vi "create backup files.vi"(8 "error in (no error)":errorcluster caption="错误输入（无错误）", 10 "execute file name":string, 11 "路径":path) -> (0 "error out":errorcluster caption="错误输出")   [LabVIEW 2016, in "数据传输系统-04.lvlib" / "update.lvlib"]
uses:
  update.lvlib
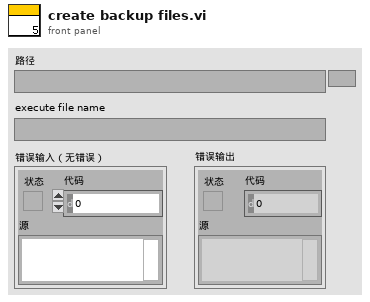
[diagram p1: front panel]
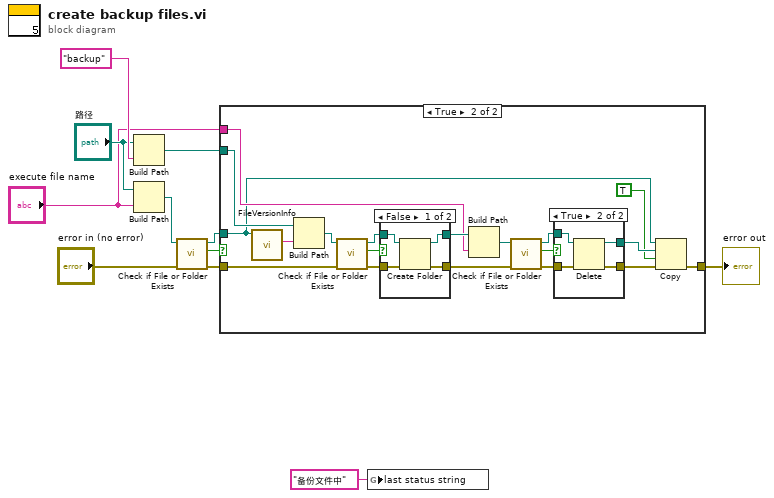
[diagram p0: block diagram]
diagram:
  n1 = Build Path(base path="路径", name or relative path="backup" ("名称或相对路径")) -> (appended path=w10:path)
  n2 = Build Path(base path="路径", name or relative path="execute file name") -> (appended path=w6:path)
  n3 = call <vilib>:"Check if File or Folder Exists.vi"("error in (no error)"="error in (no error)", "path"=w6) -> ("error out"=w3:errorcluster, "file or folder exists?"=w5:bool, "dup path"=w2:path)  [unwired: 7 in]
  n4 = case shown="True" w5 {
    tunnel: w3 -> [w12 w22]
    tunnel: w10 -> [_ w21]
    tunnel: "execute file name" -> [_ w18]
    tunnel: [w12 w14] -> w7
    tunnel: w2 -> [_ w13]
    frame False {
    }
    frame True {
      n5 = call <vilib>:"FileVersionInfo.vi"("Application Path in"=w13) -> ("File Version Info"=w20:string)  [unwired: 7 in, 3 out]
      n6 = Build Path(base path=w21, name or relative path=w20) -> (appended path=w19:path)
      n7 = call <vilib>:"Check if File or Folder Exists.vi"("error in (no error)"=w22, "path"=w19) -> ("error out"=w24:errorcluster, "file or folder exists?"=w31:bool, "dup path"=w30:path)  [unwired: 7 in]
      n8 = case shown="False" w31 {
        tunnel: w30 -> [w41 w43]
        tunnel: [w40 w43] -> w29
        tunnel: w24 -> [w39 w42]
        tunnel: [w38 w42] -> w23
        frame False {
          n9 = Create Folder(path (use dialog)=w41, error in=w39) -> (created path=w40:path, error out=w38:errorcluster)  [unwired: 1 in, 1 out]
        }
        frame True {
        }
      }
      n10 = Build Path(base path=w29, name or relative path=w18) -> (appended path=w26:path)
      n11 = call <vilib>:"Check if File or Folder Exists.vi"("error in (no error)"=w23, "path"=w26) -> ("error out"=w25:errorcluster, "file or folder exists?"=w27:bool, "dup path"=w28:path)  [unwired: 7 in]
      n12 = case shown="True" w27 {
        tunnel: w28 -> [w33 w37]
        tunnel: [w33 w36] -> w17
        tunnel: w25 -> [w32 w35]
        tunnel: [w32 w34] -> w16
        frame False {
        }
        frame True {
          n13 = Delete(path (use dialog)=w37, error in=w35) -> (deleted path=w36:path, error out=w34:errorcluster)  [unwired: 3 in, 1 out]
        }
      }
      n14 = Copy(8:w16, 9:TRUE ("覆盖(F)"), 10:w17, 11:w13) -> (0:w14:errorcluster)  [unwired: 1 in, 2 out]
    }
  }
  "error out" <- w7
  n15 = global write "更新全局变量.vi" "last status string"("备份文件中" ("last status string")) -> ()
